vi "Fire.vi"(8 "error in":errorcluster, 11 "T560Session in":refnum<class "T560Session.lvclass">) -> (0 "error out":errorcluster, 3 "T560Session out":refnum<class "T560Session.lvclass">)   [LabVIEW 2020, in "T560Session.lvclass"]
uses:
  T560Session.lvclass
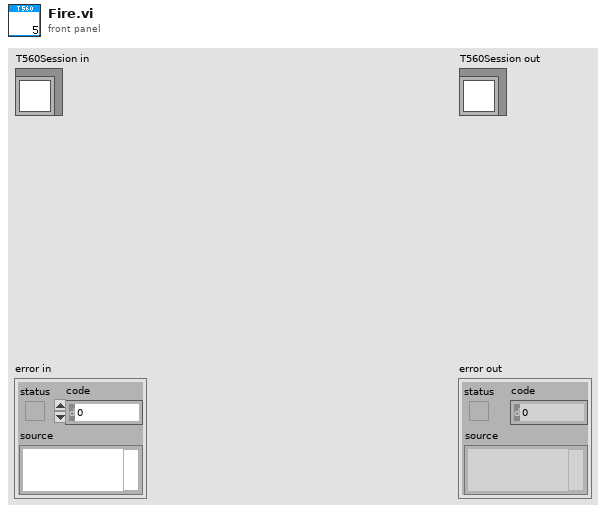
[diagram p1: front panel]
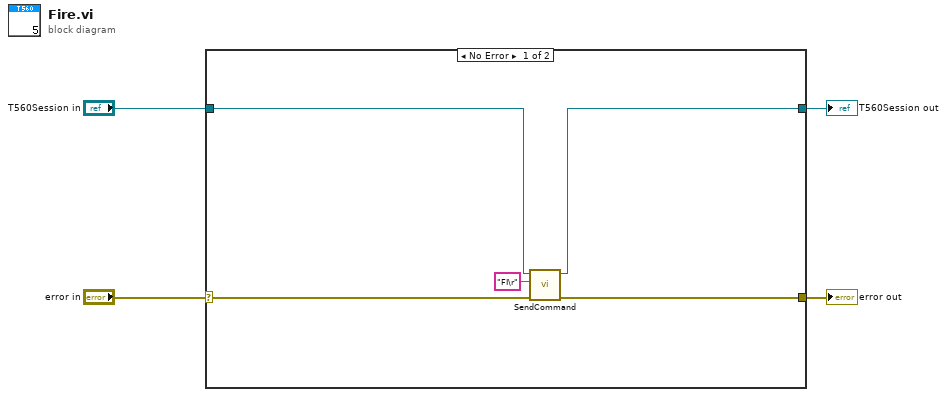
[diagram p0: block diagram]
diagram:
  n1 = case shown="No Error" "error in" {
    selector: "error in" -> [w9 w11]
    tunnel: [w8 w11] -> w3
    tunnel: [w6 w10] -> w1
    tunnel: "T560Session in" -> [w7 w10]
    frame No Error {
      n2 = call-dynamic "SendCommand.vi"("error in"=w9, "Command"="FI\r", "T560Session in"=w7) -> ("error out"=w8:errorcluster, "T560Session out"=w6:refnum<class "T560Session.lvclass">)  [unwired: 6 in, 1 out]
    }
    frame Error {
    }
  }
  "error out" <- w3
  "T560Session out" <- w1
